vi "onExecuteJob.vi"(8 "error in (no error)":errorcluster, 10 "stdin":string, 11 "Job.StaticVIRef in":refnum<class "Job.StaticVIRef.lvclass">) -> (0 "error out":errorcluster, 1 "exception":i32, 2 "stdout":string, 3 "Job.StaticVIRef out":refnum<class "Job.StaticVIRef.lvclass">)   [LabVIEW 2013, in "openCronJob.lvlib" / "Job.StaticVIRef.lvclass"]
uses:
  Job.StaticVIRef.lvclass
  Job.StaticVIRef.lvclass/Job.StaticVIRef.ctl
panel:
  # "RUNNING A JOB"
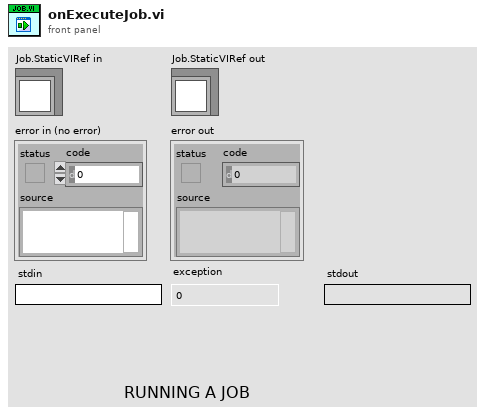
[diagram p1: front panel]
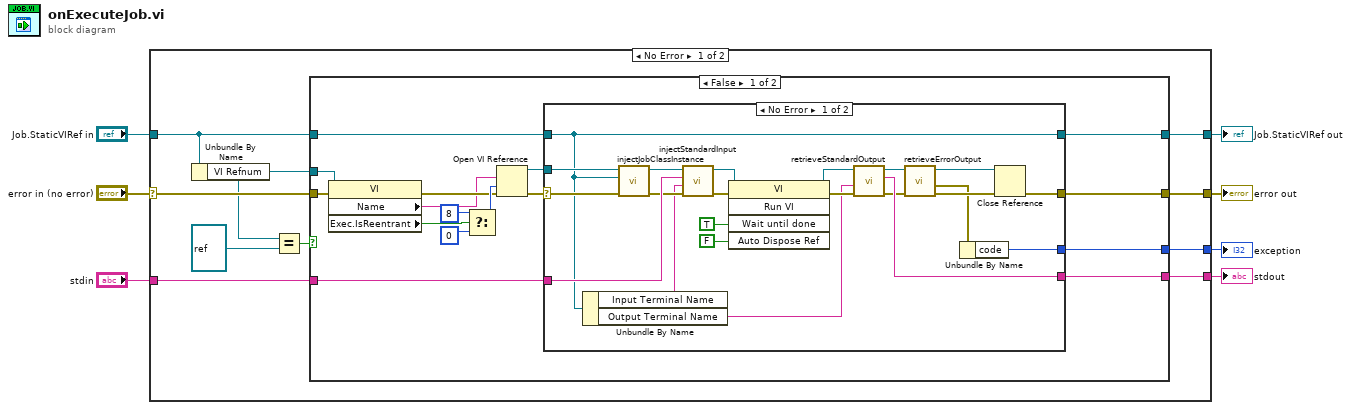
[diagram p0: block diagram]
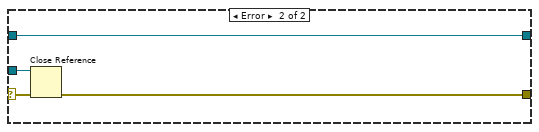
[diagram p2: hidden frame]
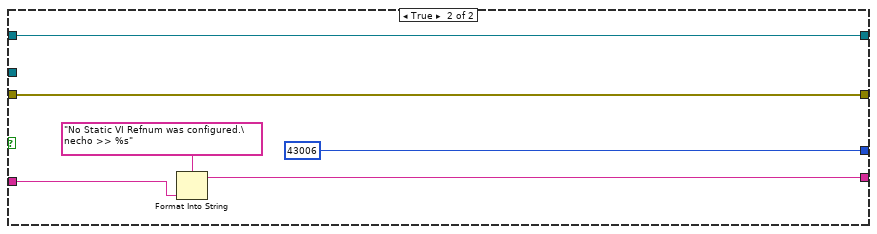
[diagram p3: hidden frame]
diagram:
  n1 = case shown="No Error" "error in (no error)" {
    selector: "error in (no error)" -> [w13 w67]
    tunnel: "stdin" -> [w17 _]
    tunnel: "Job.StaticVIRef in" -> [w8 w66]
    tunnel: [w16 _] -> w5
    tunnel: [w15 w67] -> w4
    tunnel: [w14 _] -> w3
    tunnel: [w9 w66] -> w1
    frame No Error {
      n2 = Unbundle By Name(w8) -> ("VI Refnum"=w12:refnum<vi>)
      n3 = Equal?(x=w12, y=refnum<vi> refnum) -> (x = y?=w10:bool)
      n4 = case shown="False" w10 {
        tunnel: w17 -> [w33 w64]
        tunnel: [w32 w63] -> w16
        tunnel: [w31 w62] -> w15
        tunnel: [w18 43006 ("exception")] -> w14
        tunnel: w13 -> [w23 w62]
        tunnel: w12 -> [w30 _]
        tunnel: [w19 w60] -> w9
        tunnel: w8 -> [w20 w60]
        frame False {
          n5 = property class="VI"(reference=w30, error in=w23) -> (error out=w22:errorcluster, "Name"=w21:string, "Exec.IsReentrant"=w28:bool)  [unwired: 1 out]
          n6 = Select(t=8 ("options"), s=w28, f=0 ("options")) -> (s? t:f=w26:i32)
          n7 = Open VI Reference(vi path=w21, options=w26, error in (no error)=w22) -> (vi reference=w25:refnum<vi>, error out=w24:errorcluster)  [unwired: 3 in]
          n8 = case shown="No Error" w24 {
            selector: w24 -> [w43 w57]
            tunnel: w33 -> [w53 _]
            tunnel: [w51 _] -> w32
            tunnel: [w47 w58] -> w31
            tunnel: w25 -> [w46 w59]
            tunnel: w20 -> [w38 w56]
            tunnel: [w38 w56] -> w19
            tunnel: [w34 _] -> w18
            frame No Error {
              n9 = Unbundle By Name(w38) -> ("Input Terminal Name"=w37:string, "Output Terminal Name"=w40:string)
              n10 = call "injectJobClassInstance.vi"("error in (no error)"=w43, "Job"=w38, "VI in"=w46) -> ("error out"=w44:errorcluster, "VI out"=w45:refnum<vi>)  [unwired: 7 in]
              n11 = call "injectStandardInput.vi"("error in (no error)"=w44, "control name (stdin)"=w37, "stdin"=w53, "VI in"=w45) -> ("error out"=w49:errorcluster, "VI out"=w52:refnum<vi>)  [unwired: 6 in]
              n12 = invoke class="VI" method="Run VI"(reference=w52, error in=w49, "Wait until done"=TRUE ("Wait Until Done"), "Auto Dispose Ref"=FALSE ("Auto Dispose Reference")) -> (reference out=w39:refnum<vi>, error out=w50:errorcluster)  [unwired: 1 in, 3 out]
              n13 = call "retrieveStandardOutput.vi"("error in (no error)"=w50, "control name (stdout)"=w40, "VI in"=w39) -> ("error out"=w41:errorcluster, "stdout"=w51:string, "VI out"=w42:refnum<vi>)  [unwired: 6 in]
              n14 = call "retrieveErrorOutput.vi"("error in (no error)"=w41, "VI in"=w42) -> ("error out"=w36:errorcluster, "VI Error Out"=w35:errorcluster, "VI out"=w48:refnum<vi>)  [unwired: 7 in]
              n15 = Unbundle By Name(w35) -> ("code"=w34:i32)
              n16 = Close Reference(reference=w48, error in (no error)=w36) -> (error out=w47:errorcluster)
            }
            frame Error {
              n17 = Close Reference(reference=w59, error in (no error)=w57) -> (error out=w58:errorcluster)
            }
          }
        }
        frame True {
          n18 = Format Into String(format string="No Static VI Refnum was configured.\necho >> %s", w64) -> (resulting string=w63:string)  [unwired: 2 in, 1 out]
        }
      }
    }
    frame Error {
    }
  }
  "error out" <- w4
  "Job.StaticVIRef out" <- w1
  "exception" <- w3
  "stdout" <- w5
